vi "arreglosinic.vi"(5 "dimension adqy":i32=2, 7 "dimension adqx":i32=6, 8 "DISPLONG 3":i32, 9 "DISPLONG 2":i32, 10 "DISPLONG 1":i32) -> (2 "output cluster":T1)   [LabVIEW 2016]
panel:
  in  "Cluster":T1
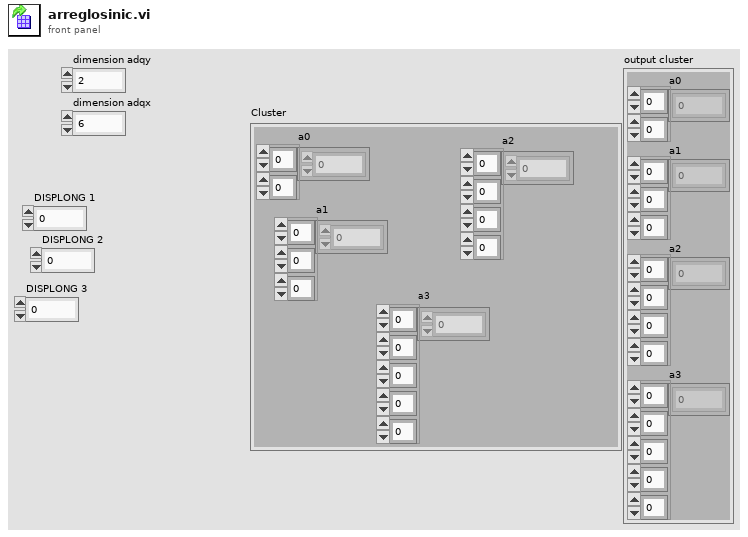
[diagram p1: front panel]
types:
  T1 = cluster{"a0":dbl[][], "a1":dbl[][][], "a2":dbl[][][][], "a3":dbl[][][][][]}
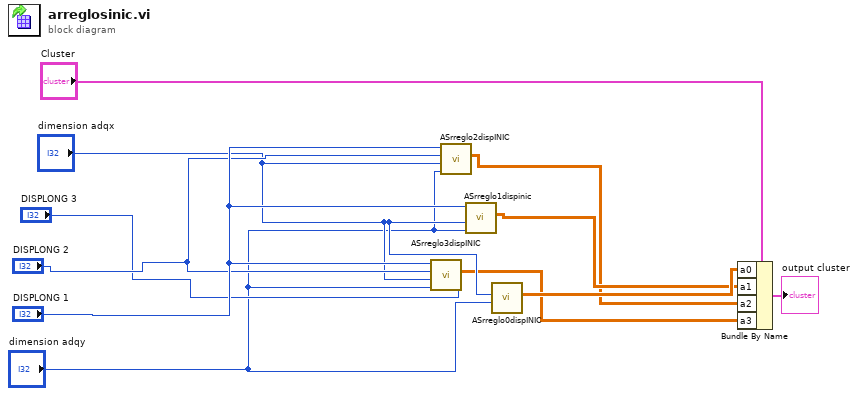
[diagram p0: block diagram]
diagram:
  n1 = call "ASrreglo3dispINIC.vi"("dimension disp 3"="DISPLONG 3", "dimension adqy"="dimension adqy", "dimension adqx"="dimension adqx", "dimension disp 2"="DISPLONG 2", "dimension disp 1"="DISPLONG 1") -> ("output array"=w2:dbl[][][][][])  [unwired: 6 in]
  n2 = call "ASrreglo2dispINIC.vi"("dimension adqy"="dimension adqy", "dimension adqx"="dimension adqx", "dimension disp 2"="DISPLONG 2", "dimension disp 1"="DISPLONG 1") -> ("output array"=w3:dbl[][][][])  [unwired: 7 in]
  n3 = call "ASrreglo1dispinic.vi"("dimension adqy"="dimension adqy", "dimension adqx"="dimension adqx", "dimension disp 1"="DISPLONG 1") -> ("output array"=w4:dbl[][][])  [unwired: 8 in]
  n4 = call "ASrreglo0dispINIC.vi"("Y"="dimension adqy", "X"="dimension adqx") -> ("output array"=w5:dbl[][])  [unwired: 9 in]
  n5 = Bundle By Name(cluster="Cluster", "a0"=w5, "a1"=w4, "a2"=w3, "a3"=w2) -> (→"output cluster":T1)
